vi "Get Target Node.vi"(8 "error in (no error)":errorcluster, 10 "Max search depth":i32, 11 "Node Ptr in":T1 format="%.0x") -> (0 "error out":errorcluster, 1 "Found?":bool, 2 "Target Ref out":refnum<k24>, 3 "Node Ptr out":T1=18446744073709551615 format="%.0x")   [LabVIEW 2019, in "TimingDRV System Explorer.lvlib"]
uses:
  TimingDRV System Explorer.lvlib
  <vilib>/NI VeriStand/Custom Device API/Custom Device Item Ref.ctl
  NationalInstruments.VeriStand.SystemDefinitionAPI
  <vilib>/NI VeriStand/Custom Device API/Custom Device API.lvlib
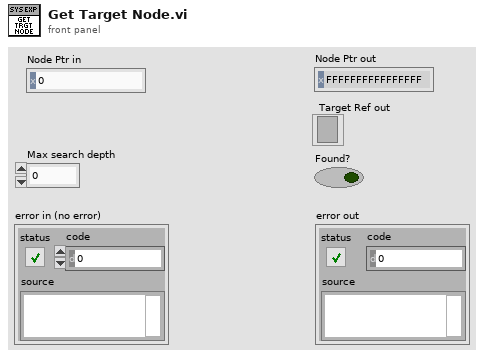
[diagram p1: front panel]
types:
  T1 = typedef "Custom Device API.lvlib/Custom Device Item Ref.ctl" = u64
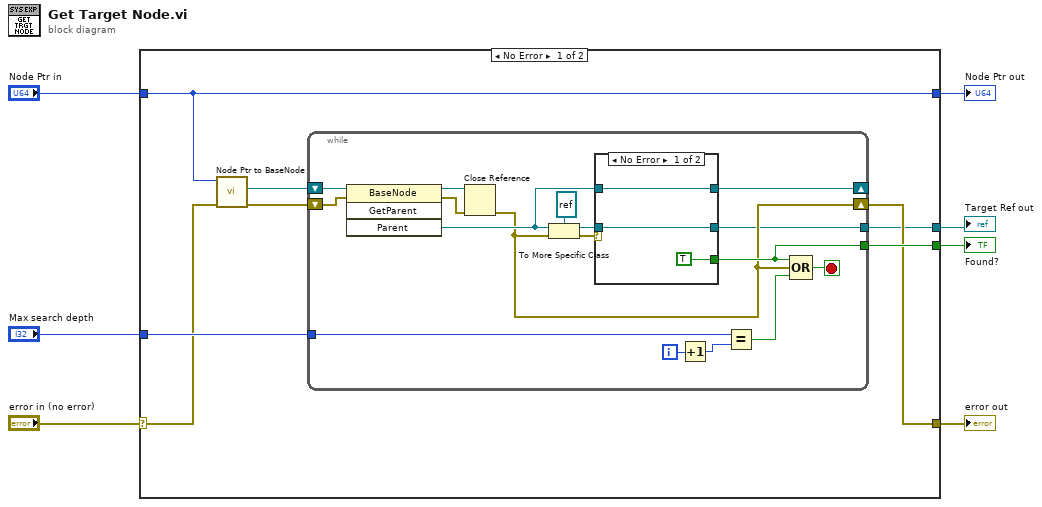
[diagram p0: block diagram]
diagram:
  n1 = case shown="No Error" "error in (no error)" {
    selector: "error in (no error)" -> [w11 w38]
    tunnel: [w14 _] -> w7
    tunnel: "Max search depth" -> [w13 _]
    tunnel: "Node Ptr in" -> [w9 w37]
    tunnel: [w10 w38] -> w3
    tunnel: [w9 w37] -> w2
    tunnel: [w8 _] -> w1
    frame No Error {
      n2 = call "Node Ptr to BaseNode.vi"("error in (no error)"=w11, "nodeID in"=w9) -> ("error out"=w15:errorcluster, ".NET Refnum out"=w12:refnum<k24>)  [unwired: 7 in, 1 out]
      n3 = while {
        shift-right: [w28] -> _
        shift-left: w12 -> [w32]
        tunnel: w13 -> [w26]
        tunnel: [w22] -> w14
        shift-right: [w18] -> w10
        shift-left: w15 -> [w21]
        tunnel: [w16] -> w8
        i -> [w25]
        stop <- w27 stop-if-true
        n4 = invoke class="BaseNode" method="GetParent"(reference=w32, error in=w21) -> (reference out=w19:refnum<k24>, error out=w20:errorcluster, "Parent"=w29:refnum<k24>)  [unwired: 2 in, 1 out]
        n5 = Close Reference(reference=w19, error in (no error)=w20) -> (error out=w18:errorcluster)
        n6 = To More Specific Class(target class=refnum<k24> refnum ("element"), reference=w29, error in=w18) -> (specific class reference=w17:refnum<k24>, error out=w30:errorcluster)
        n7 = case shown="No Error" w30 {
          tunnel: w29 -> [w35 w36]
          tunnel: [w35 w36] -> w28
          tunnel: [TRUE _] -> w22
          tunnel: w17 -> [w33 _]
          tunnel: [w33 _] -> w16
          frame No Error {
          }
          frame Error {
          }
        }
        n8 = Increment(x=w25) -> (x+1=w24:i32)
        n9 = Equal?(x=w26, y=w24) -> (x = y?=w23:bool)
        n10 = Compound Arithmetic op=OR(w22, w18, w23) -> (w27:bool)
      }
    }
    frame Error {
    }
  }
  "Found?" <- w7
  "error out" <- w3
  "Node Ptr out" <- w2
  "Target Ref out" <- w1
